vi "run_ICov_tests.vi"(8 "error in (no error)":errorcluster, 10 "<<Unit test folder>>":path=path "C:/git/instacoverage/2018/Providers/InstaCoverage", 11 "<<UnitTest project path>>":path=path "C:/git/instacoverage/2018/Providers/InstaCoverage/UnitTest.lvproj") -> (0 "error out":errorcluster)   [LabVIEW 2018]
uses:
  <resource>/Framework/Providers/InstaCoverage/Core/Defines/TestReportTypeEnum.ctl
  <resource>/Framework/Providers/InstaCoverage/Core/InstaCoverageCore.lvlib
  <resource>/Framework/Providers/InstaCoverage/Pro/InstaCoveragePro.lvlib
  <resource>/Framework/Providers/InstaCoverage/Core/Defines/CoverageResult.ctl
  <resource>/Framework/Providers/InstaCoverage/Core/TestSuite/TestSuite.lvclass
panel:
  out "error message":string
  out "Exit code":i32
  in  "arguments":string[](array[string])
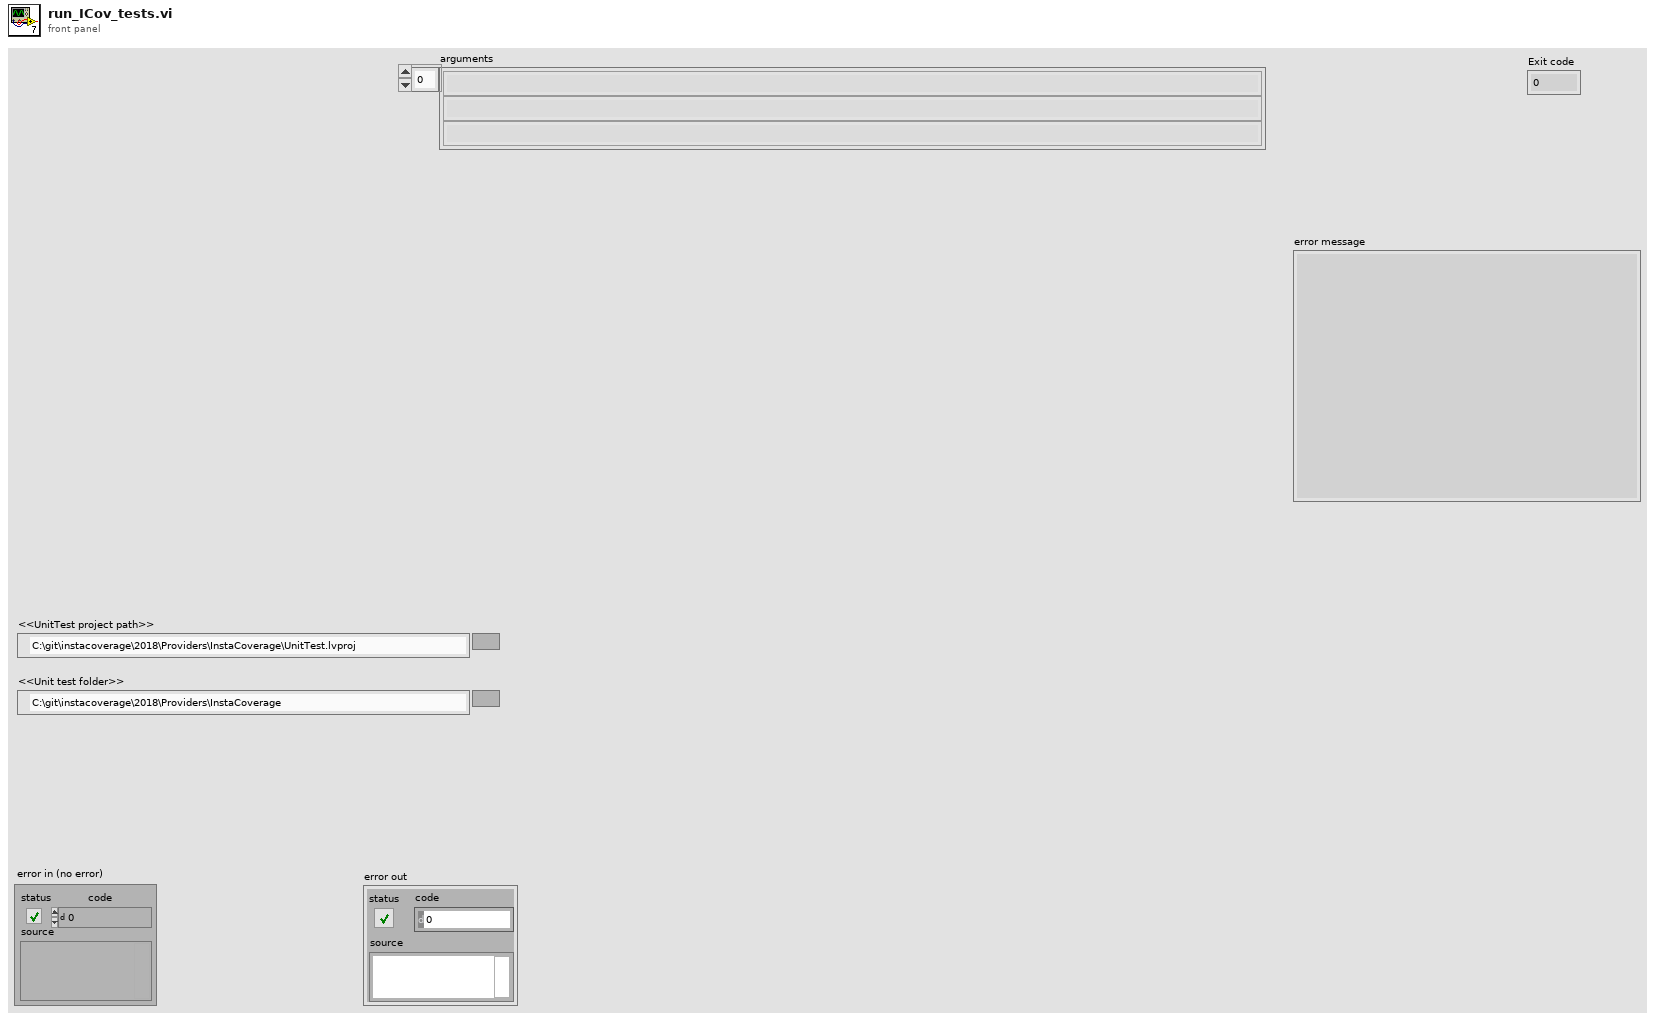
[diagram p1: front panel]
types:
  T1 = typedef "InstaCoverage.lvlib/InstaCoverageCore.lvlib/TestReportTypeEnum.ctl" = enum16{"JUNIT_XML", "HTML"}
  T2 = typedef "InstaCoverage.lvlib/InstaCoverageCore.lvlib/CoverageResult.ctl" = enum16{"100%", "NOT 100%", "N/A", "AVAILABLE IN PRO"}
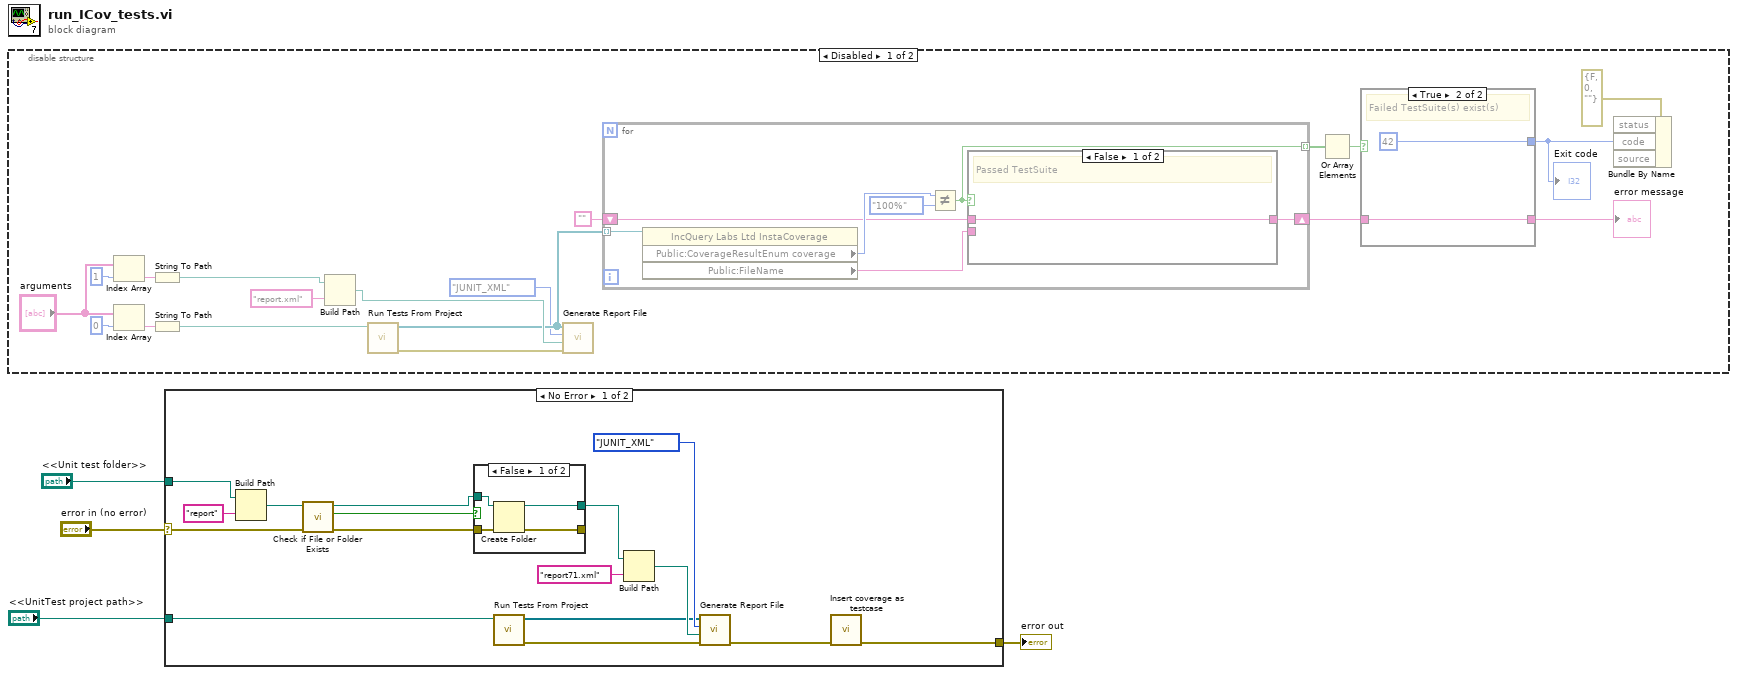
[diagram p0: block diagram]
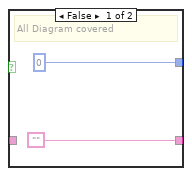
[diagram p2: hidden frame]
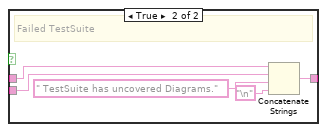
[diagram p3: hidden frame]
diagram:
  n1 = disable-structure shown="Disabled" {
    frame Disabled {
      n2 = Index Array(array="arguments", index=1) -> (element=w19:string)
      n3 = Index Array(array="arguments", index=0) -> (element=w21:string)
      n4 = String To Path(string=w19) -> (path=w16:path)
      n5 = String To Path(string=w21) -> (path=w17:path)
      n6 = Build Path(base path=w16, name or relative path="report.xml") -> (appended path=w23:path)
      n7 = call <resource>:"Run Tests From Project.vi"("Path lvProject"=w17) -> ("Error out"=w9:errorcluster, "TestSuite[] results"=w15:refnum<class "TestSuite.lvclass">[])  [unwired: 9 in]
      n8 = call <resource>:"Generate Report File.vi"("Error In"=w9, "Path reportFile"=w23, "TestReportTypeEnum in"=TestReportTypeEnum."JUNIT_XML", "TestSuite[] in"=w15) -> ()  [unwired: 7 in, 1 out]
      n9 = for {
        tunnel: w15 -> [w32] mode=indexing
        tunnel: [w31] -> w14 mode=indexing
        shift-right: [w28] -> w11
        shift-left: "" -> [w30]
        n10 = property class="IncQuery Labs Ltd InstaCoverage"(reference=w32) -> ("Public:CoverageResultEnum coverage"=w34:T2, "Public:FileName"=w29:string)  [unwired: 1 in, 2 out]
        n11 = Not Equal?(x=w34, y=CoverageResult."100%") -> (x != y?=w31:bool)
        n12 = case shown="False" w31 {
          tunnel: w30 -> [w35 w39]
          tunnel: w29 -> [_ w38]
          tunnel: [w35 w40] -> w28
          frame False {
            # "Passed TestSuite"
          }
          frame True {
            # "Failed TestSuite"
            n13 = Concatenate Strings(w39, w38, " TestSuite has uncovered Diagrams." ("string"), "\n") -> (w40:string)
          }
        }
      }
      n14 = Or Array Elements(Boolean array=w14) -> (logical OR=w13:bool)
      n15 = case shown="True" w13 {
        tunnel: [0 ("Exit code") 42 ("Exit code")] -> w5
        tunnel: ["" w26] -> w12
        tunnel: w11 -> [_ w26]
        frame False {
          # "All Diagram covered"
        }
        frame True {
          # "Failed TestSuite(s) exist(s)"
        }
      }
      "Exit code" <- w5
      "error message" <- w12
      n16 = Bundle By Name(cluster=errorcluster {"status"=FALSE, "code"=0, "source"=""} ("error out"), "code"=w5) -> ()  [unwired: 2 in, 1 out]
    }
    frame Enabled {
    }
  }
  n17 = case shown="No Error" "error in (no error)" {
    selector: "error in (no error)" -> [w49 w63]
    tunnel: "<<UnitTest project path>>" -> [w44 _]
    tunnel: "<<Unit test folder>>" -> [w50 _]
    tunnel: [w41 w63] -> w1
    frame No Error {
      n18 = Build Path(base path=w50, name or relative path="report") -> (appended path=w56:path)
      n19 = call <vilib>:"Check if File or Folder Exists.vi"("error in (no error)"=w49, "path"=w56) -> ("error out"=w53:errorcluster, "file or folder exists?"=w55:bool, "dup path"=w54:path)  [unwired: 7 in]
      n20 = case shown="False" w55 {
        tunnel: w54 -> [w60 w62]
        tunnel: [w59 w62] -> w48
        tunnel: w53 -> [w58 w61]
        tunnel: [w57 w61] -> _
        frame False {
          n21 = Create Folder(path (use dialog)=w60, error in=w58) -> (created path=w59:path, error out=w57:errorcluster)  [unwired: 1 in, 1 out]
        }
        frame True {
        }
      }
      n22 = call <resource>:"Run Tests From Project.vi"("Path lvProject"=w44) -> ("Error out"=w47:errorcluster, "TestSuite[] results"=w43:refnum<class "TestSuite.lvclass">[])  [unwired: 9 in]
      n23 = Build Path(base path=w48, name or relative path="report71.xml") -> (appended path=w46:path)
      n24 = call <resource>:"Generate Report File.vi"("Error In"=w47, "Path reportFile"=w46, "TestReportTypeEnum in"=TestReportTypeEnum."JUNIT_XML", "TestSuite[] in"=w43) -> ("Error Out"=w42:errorcluster)  [unwired: 7 in]
      n25 = call "Insert coverage as testcase.vi"("Error in"=w42) -> ("error out"=w41:errorcluster)  [unwired: 10 in]
    }
    frame Error {
    }
  }
  "error out" <- w1
